vi "Filter 2(SubVI).vi"(10 "NewVal":dbl, 11 "OldVal":dbl) -> (3 "Val":dbl)   [LabVIEW 2017]
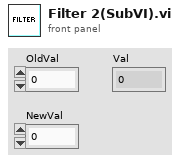
[diagram p1: front panel]
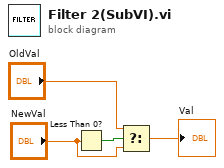
[diagram p0: block diagram]
diagram:
  n1 = Less Than 0?(x="NewVal") -> (x < 0?=w4:bool)
  n2 = Select(t="OldVal", s=w4, f="NewVal") -> (s? t:f=→"Val":dbl)
